vi "8) While Loop.vi"() -> ()   [LabVIEW 2018]
panel:
  in  "milliseconds to wait":u32
  in  "stop":bool
  in  "Temperature (F)":dbl(slide) scale=0.0..100.0
  out "Temperature (C)":dbl(slide) scale=0.0..100.0
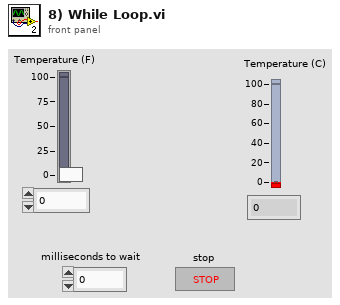
[diagram p1: front panel]
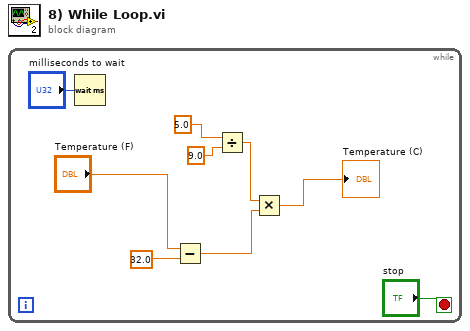
[diagram p0: block diagram]
diagram:
  n1 = while {
    stop <- "stop" stop-if-true
    n2 = Wait (ms)(milliseconds to wait="milliseconds to wait") -> ()  [unwired: 1 out]
    n3 = Subtract(x="Temperature (F)", y=32.0 ("x-y")) -> (x-y=w8:dbl)
    n4 = Divide(x=5.0 ("x/y"), y=9.0) -> (x/y=w9:dbl)
    n5 = Multiply(x=w9, y=w8) -> (x*y=→"Temperature (C)":dbl)
  }
